vi "GCMPlugin_IsSupportingItem.vi"(8 "error in (no error)":errorcluster, 9 "VI Reference":refnum<vi>, 10 "ProjectItem Refnum":refnum<vi>, 11 "_ClassRenamer in":refnum<class "ClassRenamer.lvclass">) -> (0 "error out":errorcluster, 2 "IsSupportingItem":bool, 3 "_ClassRenamer out":refnum<class "ClassRenamer.lvclass">)   [LabVIEW 2014, in "ClassRenamer.lvclass"]
uses:
  ClassRenamer.lvclass
  GCMCore/Providers/Veritech_GCM/Support/Utilites/_ProjectItemsUtilities/_ProjectItemsUtilities.lvlib
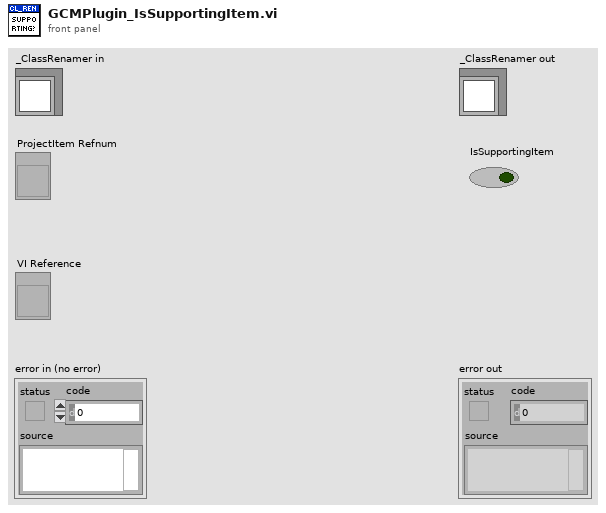
[diagram p1: front panel]
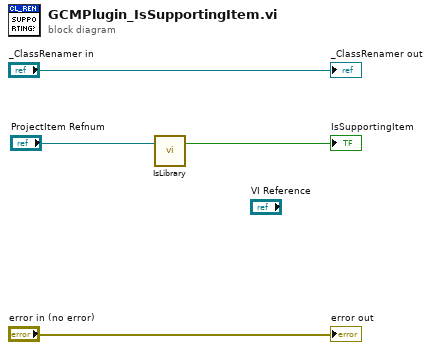
[diagram p0: block diagram]
diagram:
  n1 = call "IsLibrary.vi"("ProjectItem Refnum"="ProjectItem Refnum") -> ("IsLibrary?"=→"IsSupportingItem":bool)  [unwired: 2 in]
  "error out" <- "error in (no error)"
  "_ClassRenamer out" <- "_ClassRenamer in"
